vi "CameraQueryAcquire.vi"(8 "error in (no error)":errorcluster, 11 "CameraBase in":refnum<class "CameraBase.lvclass">) -> (0 "error out":errorcluster, 1 "frames":u32, 2 "acquiring":bool, 3 "CameraBase out":refnum<class "CameraBase.lvclass">)   [LabVIEW 2012, in "CameraBase.lvclass"]
doc: "Returns an array of camera communicated with by this SDK"
uses:
  <userlib>/BIAS2/classes/CameraBase/CameraBase.lvclass
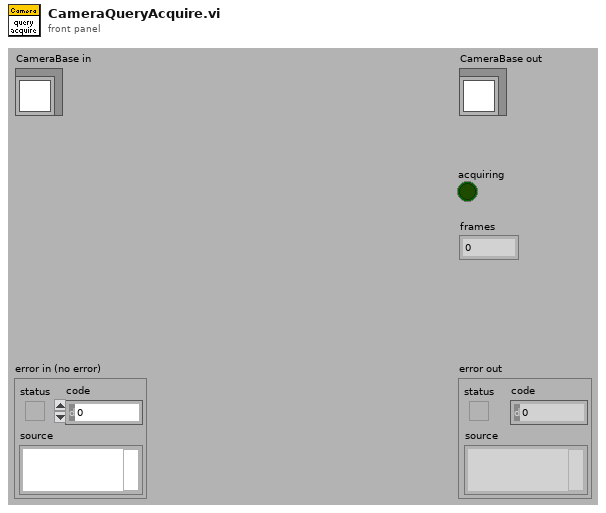
[diagram p1: front panel]
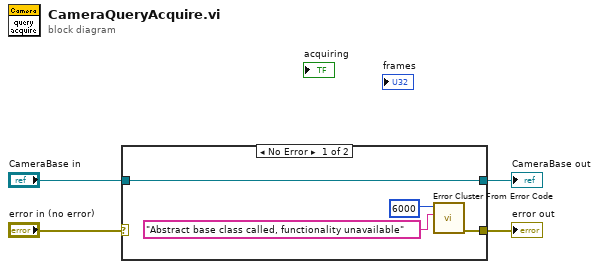
[diagram p0: block diagram]
diagram:
  n1 = case shown="No Error" "error in (no error)" {
    selector: "error in (no error)" -> [_ w10]
    tunnel: [w6 w10] -> w3
    tunnel: [w8 w9] -> w1
    tunnel: "CameraBase in" -> [w8 w9]
    frame No Error {
      n2 = call <vilib>:"Error Cluster From Error Code.vi"("error message (\"\")"="Abstract base class called, functionality unavailable" ("format string"), "error code (0)"=6000) -> ("error out"=w6:errorcluster)  [unwired: 7 in]
    }
    frame Error {
    }
  }
  "error out" <- w3
  "CameraBase out" <- w1
